vi "Read Incoming Bytes.vi"(8 "error in (no error)":errorcluster, 9 "timeout (1000 ms)":i32=1000, 10 "max bytes to read (100000)":i32=100000, 11 "Connection.Collection":refnum<class "Connection.Collection.lvclass">) -> (0 "error out":errorcluster, 1 "timed out":bool, 2 "Bytes":u8[](array[numeric]) format="%08b", 3 "Connection.Collection":refnum<class "Connection.Collection.lvclass">, 4 "connected":bool)   [LabVIEW 2013, in "Connection_GOSPL.lvlib" / "Connection.Collection.lvclass"]
uses:
  Connection.Collection.lvclass
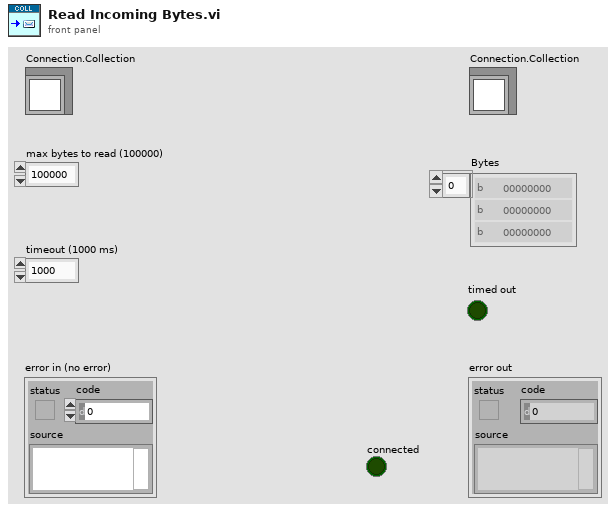
[diagram p1: front panel]
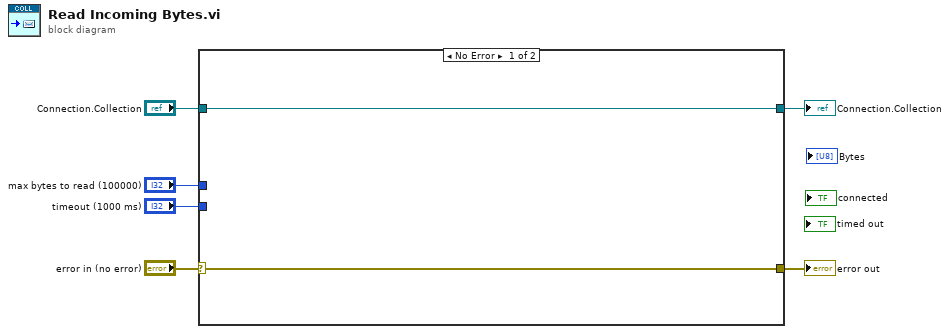
[diagram p0: block diagram]
diagram:
  n1 = case shown="No Error" "error in (no error)" {
    selector: "error in (no error)" -> [w8 w10]
    tunnel: [w8 w10] -> w5
    tunnel: [w7 w9] -> w3
    tunnel: "Connection.Collection" -> [w7 w9]
    tunnel: "max bytes to read (100000)" -> [_ _]
    tunnel: "timeout (1000 ms)" -> [_ _]
    frame No Error {
    }
    frame Error {
    }
  }
  "error out" <- w5
  "Connection.Collection" <- w3
